vi "Set Pin Map ID.vi"(8 "error in":errorcluster, 10 "Sequence Context":refnum<k7>, 11 "pin_map_id":string) -> (0 "error out":errorcluster)   [LabVIEW 2020, in "NIDCPowerSourceDCVoltage.lvlib"]
uses:
  NIDCPowerSourceDCVoltage.lvlib
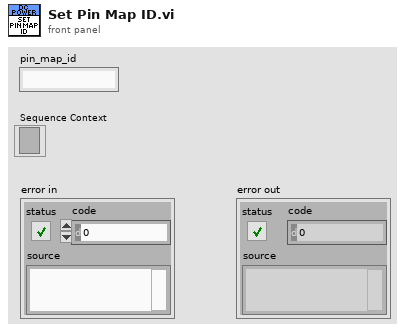
[diagram p1: front panel]
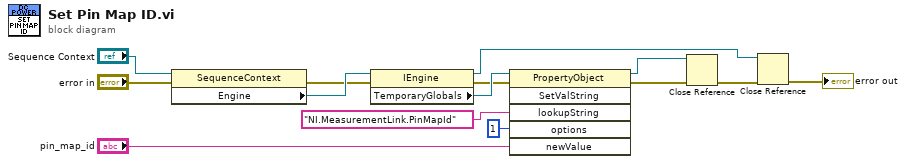
[diagram p0: block diagram]
diagram:
  n1 = property class="SequenceContext"(reference="Sequence Context", error in="error in") -> (error out=w4:errorcluster, "Engine"=w6:refnum<k7>)  [unwired: 1 out]
  n2 = property class="IEngine"(reference=w6, error in=w4) -> (reference out=w12:refnum<k7>, error out=w2:errorcluster, "TemporaryGlobals"=w7:refnum<k7>)
  n3 = invoke class="PropertyObject" method="SetValString"(reference=w7, error in=w2, "lookupString"="NI.MeasurementLink.PinMapId", "options"=1, "newValue"="pin_map_id") -> (reference out=w10:refnum<k7>, error out=w11:errorcluster)  [unwired: 1 in, 4 out]
  n4 = Close Reference(reference=w10, error in (no error)=w11) -> (error out=w13:errorcluster)
  n5 = Close Reference(reference=w12, error in (no error)=w13) -> (error out=→"error out":errorcluster)
